vi "Error Global.vi"() -> ()   [LabVIEW 2021, in "CIFCorePlugin.lvclass"]
uses:
  CIFCorePlugin.lvclass
panel:
  in  "Config Parse Error":errorcluster={"status"=FALSE, "code"=-8002, "source"="The JSON string received over gRPC could not be parsed to update the configuration. Check the JSON string.  Received string: \n "}
  in  "gRPC Server Not Found":errorcluster={"status"=TRUE, "code"=-8001, "source"="gRPC Server was not found in the MAP.  Check that the proper class was wired in to search and that the class was already registered in the MAP. "}
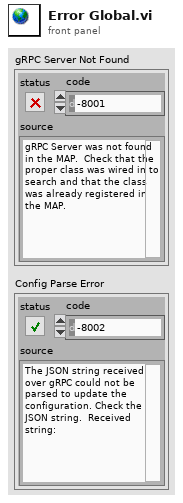
[diagram p1: front panel]
diagram:
